vi "Stop Services.vi"(8 "error in (no error)":errorcluster, 10 "count services":i32, 11 "Manejo Turnos in":refnum<class "Manejo Turnos.lvclass">) -> (0 "error out":errorcluster, 3 "Manejo Turnos out":refnum<class "Manejo Turnos.lvclass">)   [LabVIEW 2020, in "Manejo Turnos.lvlib" / "Manejo Turnos.lvclass"]
uses:
  Manejo Turnos.lvclass
  Manejo Turnos.lvclass/Manejo Turnos.ctl
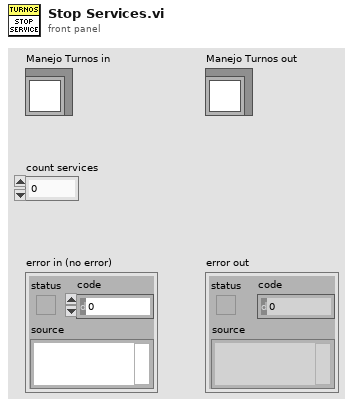
[diagram p1: front panel]
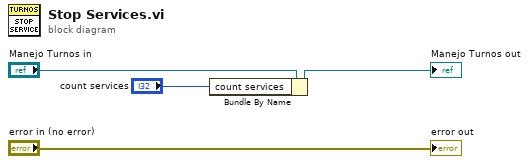
[diagram p0: block diagram]
diagram:
  n1 = Bundle By Name(cluster="Manejo Turnos in", "count services"="count services") -> (→"Manejo Turnos out":refnum<class "Manejo Turnos.lvclass">)
  "error out" <- "error in (no error)"
